vi "AlazarBeforeAsyncRead.vi"(0 "Handle":u32, 1 "Channel":u32(ring)=1 items=["A"=1, "B"=2, "A + B"=3, "C"=4, "A + C"=5, "A + B"=6, "D"=8, "A + D"=9, "B + D"=10, "C + D"=12, "A + B + C + D"=15], 2 "Offset":u32, 3 "Length":u32, 4 "Records Per Buffer":u32, 5 "Records Count":u32, 6 "cFlags":u32, 7 "error in (no error)":errorcluster) -> (20 "Handle":u32, 26 "Return Code":u32, 27 "error out":errorcluster)   [LabVIEW 2024]
doc: "Configure a board to make an asynchronous AutoDMA acquisition."
uses:
  ATSApi.dll
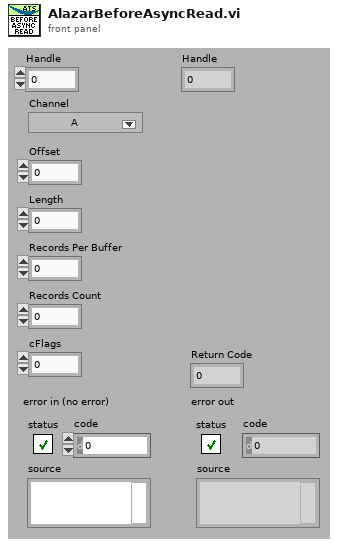
[diagram p1: front panel]
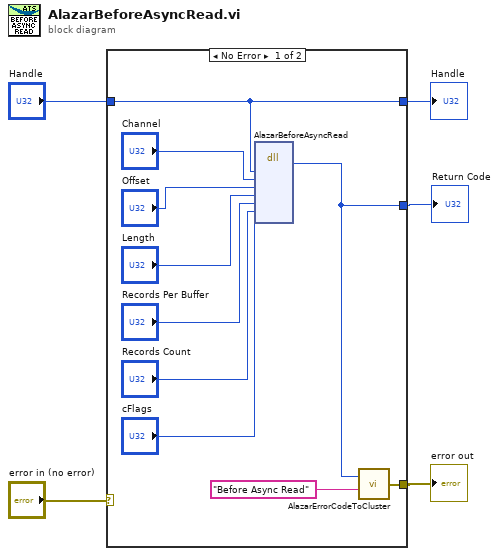
[diagram p0: block diagram]
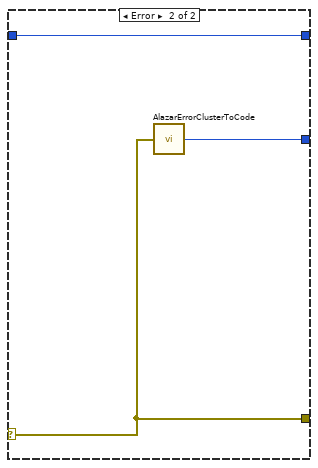
[diagram p2: hidden frame]
diagram:
  n1 = case shown="No Error" "error in (no error)" {
    selector: "error in (no error)" -> [_ w18]
    tunnel: [w13 w18] -> w4
    tunnel: [w15 w17] -> w3
    tunnel: "Handle" -> [w12 w16]
    tunnel: [w12 w16] -> w1
    frame No Error {
      n2 = dll-call lib="ATSApi.dll" fn="AlazarBeforeAsyncRead"("handle"=w12, "channelSelect"="Channel", "transferOffset"="Offset", "transferLength"="Length", "recordsPerBuffer"="Records Per Buffer", "recordsCount"="Records Count", "cFlags"="cFlags") -> (w15:u32)  [unwired: 10 in, 2 out]
      n3 = call "AlazarErrorCodeToCluster.vi"("Message"="Before Async Read", "Error Code"=w15) -> ("error out"=w13:errorcluster)
    }
    frame Error {
      n4 = call "AlazarErrorClusterToCode.vi"("error in (no error)"=w18) -> ("Error Code"=w17:u32)
    }
  }
  "Handle" <- w1
  "error out" <- w4
  "Return Code" <- w3
